vi "move_back.vi"(1 "Ant's memory":u8[](array[numeric])) -> (0 "action":T1)   [LabVIEW 2015]
uses:
  ant_base/action_cluster.ctl
  ant_base/actionType_enum.ctl
  ant_base/ant_base.lvclass
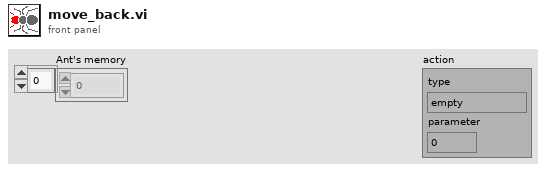
[diagram p1: front panel]
types:
  T1 = typedef "ant_base.lvclass/action_cluster.ctl" = cluster{"type":T2, "parameter":dbl}
  T2 = typedef "ant_base.lvclass/actionType_enum.ctl" = enum8{"empty", "move", "take", "put", "mark"}
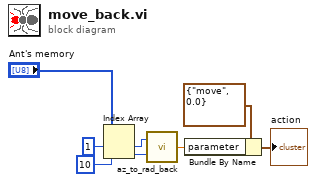
[diagram p0: block diagram]
diagram:
  n1 = Index Array(array="Ant's memory", index #1=1 ("index"), index #2=10 ("index")) -> (element #1=w3:u8, element #2=w2:u8)
  n2 = call "az_to_rad_back.vi"("az quantity"=w2, "az"=w3) -> ("rad"=w1:dbl)
  n3 = Bundle By Name(cluster=T1 {"type"=enum."move", "parameter"=0.0} ("action"), "parameter"=w1) -> (→"action":T1)
